vi "Read Configuration File Path.vi"(8 "error in (no error)":errorcluster, 11 "Configuration in":refnum<class "Configuration.lvclass">) -> (0 "error out":errorcluster, 2 "Configuration File Path":path, 3 "Configuration out":refnum<class "Configuration.lvclass">)   [LabVIEW 2017, in "Configuration.lvlib" / "Configuration.lvclass"]
uses:
  Configuration.lvclass
  Configuration.lvclass/Configuration.ctl
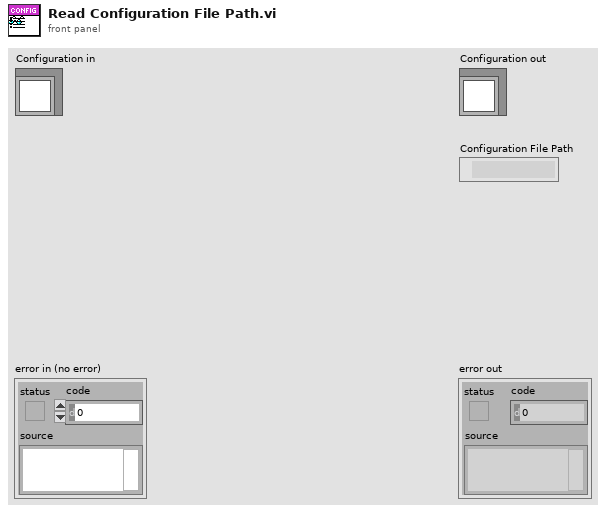
[diagram p1: front panel]
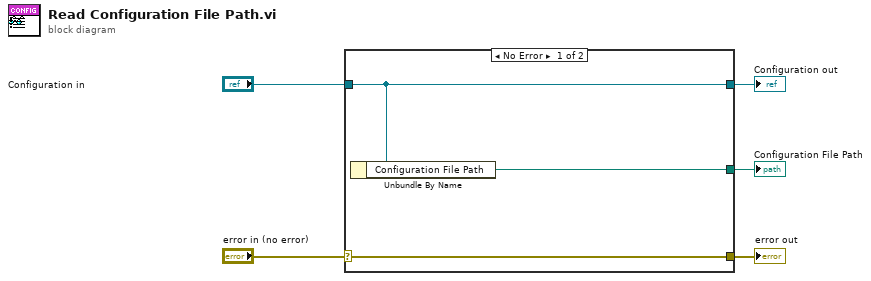
[diagram p0: block diagram]
diagram:
  n1 = case shown="No Error" "error in (no error)" {
    selector: "error in (no error)" -> [w8 w9]
    tunnel: [w8 w9] -> w4
    tunnel: [w7 w10] -> w2
    tunnel: "Configuration in" -> [w7 w10]
    tunnel: [w6 _] -> w1
    frame No Error {
      n2 = Unbundle By Name(w7) -> ("Configuration File Path"=w6:path)
    }
    frame Error {
    }
  }
  "error out" <- w4
  "Configuration out" <- w2
  "Configuration File Path" <- w1
